vi "LIDAR Debug Platform.vi"() -> ()   [LabVIEW 2009]
uses:
  <vilib>/rvi/interface/nirviOpenFPGA/nirviOpenFPGA.xnode
  FPGA Bitfiles/Athena Brain.lvproj_FPGA Target 2_serial FPGA Main.vi.lvbitx
  serial FPGA Main.vi
  <vilib>/FPGAPlugInAG/sbRIO-9642/nirviIntfOpen_sbRIO-9642.vi
  <vilib>/rvi/interface/nirviMethod/nirviMethod.xnode
  <vilib>/rvi/interface/common/niFpgaNodeNameForErrorReporting.ctl
  <vilib>/rvi/errors/niLvFpgaWhatHappensToTopLevelVI.ctl
  <vilib>/Utility/error.llb/Error Cluster From Error Code.vi
  <vilib>/RVI Host/nirviSupport.llb/nirviErrorClusterFromErrorCode.vi
  <vilib>/LabVIEW Targets/FPGA/RIO/nirio_HostInterface/nirio_EnableInterrupts.vi
  <vilib>/rvi/errors/niLvFpgaReportInternalErrorWithAdditionalInfo.vi
  <vilib>/rvi/errors/niLvFpgaAdjustHostInterfaceError.vi
  FPGA/behaviors/driveable path/drivable paths global.vi
  <vilib>/userDefined/High Color/nirio_resource_hc.ctl
  NiRioSrv.dll
  <vilib>/rvi/FIFO/Fifo_Resource/nirvififoUniquifyingName.vi
  <vilib>/rvi/DataTransferAndStorage/Container/XNode/niFpgaContainer.xnode
panel:
  out "process time":u32
  out "transform":u32
  out "XY Graph":T1(graph)
  in  "write?":bool
  in  "Data to write":string="\u0002\u0000\u0002\u0000 $4\b"
  out "error out":errorcluster
  out "LIDAR String":string
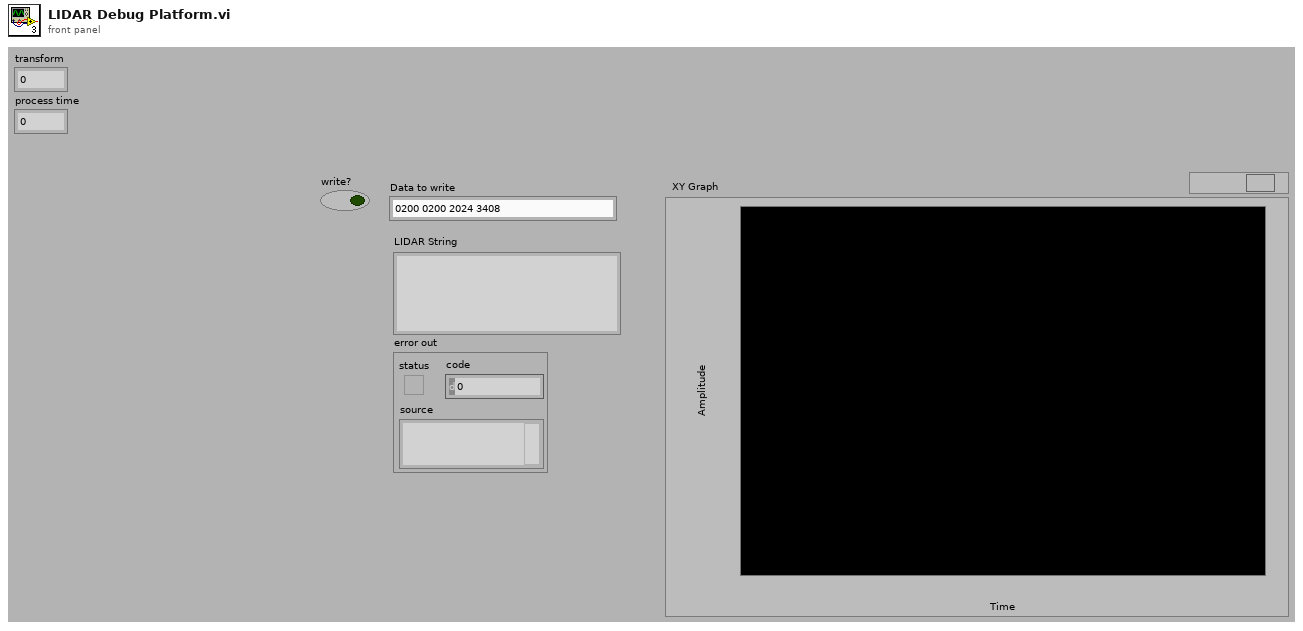
[diagram p1: front panel]
types:
  T1 = cluster{"New X Position":i16, "New Y Position":i16}[]
  T2 = typedef "serial FPGA main reference type def.ctl" = refnum<k20>
  T3 = enum16{"confirm check sum", "check status byte", "read measured values", "confirm measurement", "confirm command", "read message length", "read address", "wait for \"02\""}
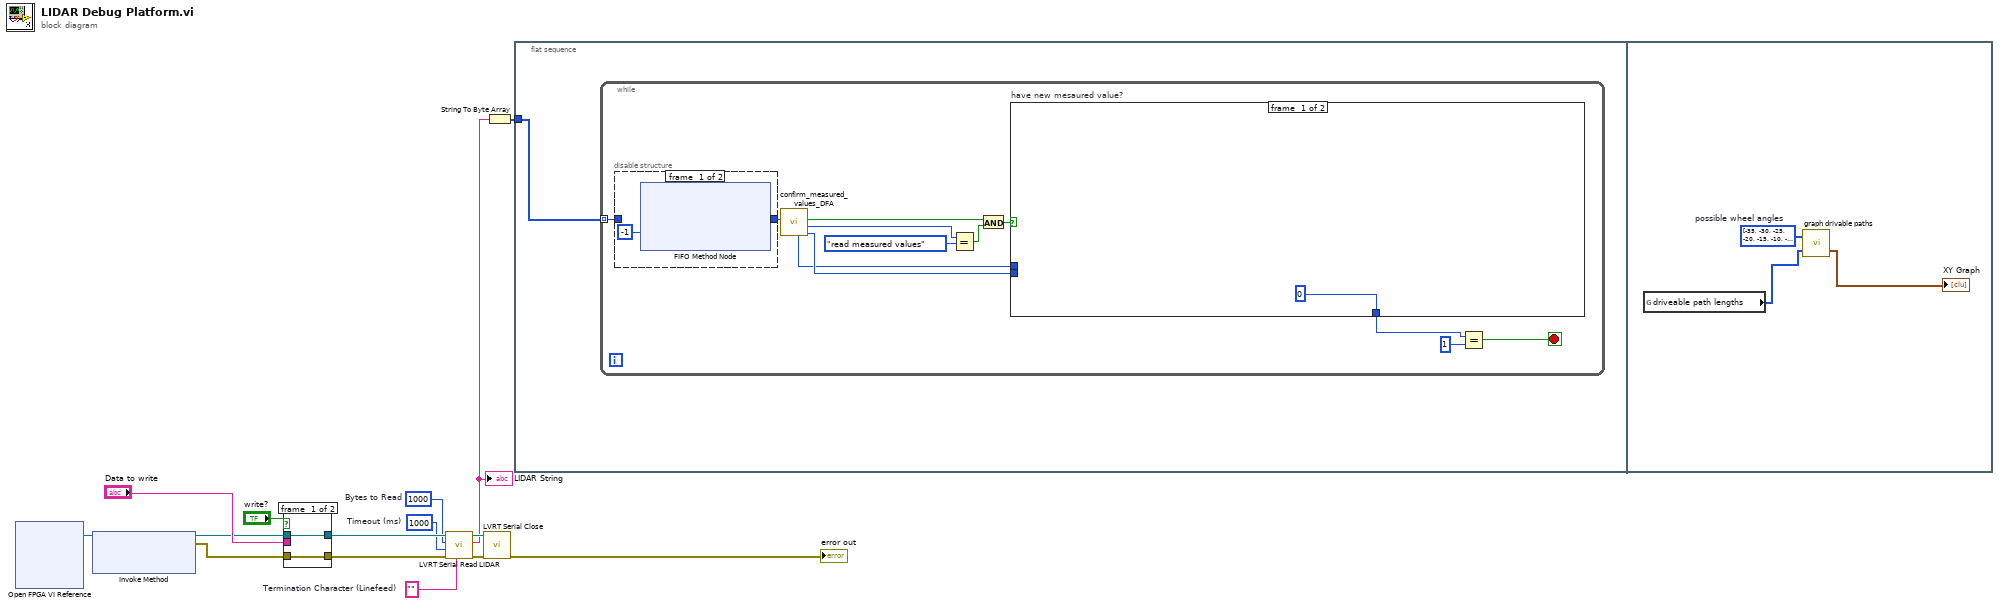
[diagram p0: block diagram]
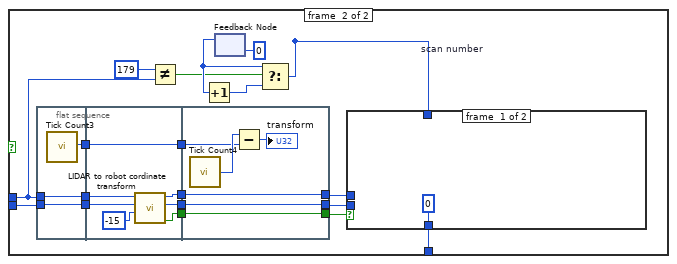
[diagram p3: hidden frame]
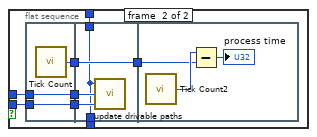
[diagram p4: hidden frame]
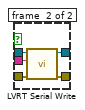
[diagram p5: hidden frame]
diagram:
  w5 = ""  # Termination Character (Linefeed)
  w10 = 1000  # Timeout (ms)
  w12 = u32 1000  # Bytes to Read
  n1 = xnode "Open FPGA VI Reference"() -> ("FPGA VI Reference Out"=w8:refnum<k20>)  [unwired: 2 in, 1 out]
  n2 = xnode "Invoke Method"("FPGA VI Reference In"=w8) -> ("FPGA VI Reference Out"=w7:refnum<k20>, "error out"=w6:errorcluster)  [unwired: 1 in, 1 out]
  n3 = case shown="False" "write?" {
    tunnel: "Data to write" -> [_ w22]
    tunnel: [w16 w21] -> w14
    tunnel: [w17 w20] -> w13
    tunnel: w7 -> [w17 w19]
    tunnel: w6 -> [w16 w18]
    frame #0 {
    }
    frame #1 {
      n4 = call "LVRT Serial Write.vi"("error in (no error)"=w18, "String"=w22, "FPGA Main Ref"=w19) -> ("error out"=w21:errorcluster, "FPGA Main Ref Out"=w20:T2)  [unwired: 7 in]
    }
  }
  n5 = call "LVRT Serial Read LIDAR.vi"("Termination Character (Linefeed)"=w5, "error in (no error)"=w14, "Timeout (ms) (-1: no timeout)"=w10, "Bytes to Read"=w12, "FPGA Main Ref"=w13) -> ("error out"=w4:errorcluster, "LIDAR"=w2:string, "FPGA Main Ref Out"=w3:T2)  [unwired: 4 in]
  "LIDAR String" <- w2
  n6 = call "LVRT Serial Close.vi"("error out"=w4, "FPGA Main Ref"=w3) -> ("error out"=→"error out":errorcluster)  [unwired: 9 out]
  n7 = String To Byte Array(string=w2) -> (unsigned byte array=w1:u8[])
  n8 = flat-sequence {
    tunnel: w1 -> [w23]
    frame #0 {
      n9 = while {
        tunnel: w23 -> [w28] mode=indexing
        stop <- w24 stop-if-true
        n10 = disable-structure shown="Enabled" {
          disable-tunnel: [w37 w86] -> w35
          disable-tunnel: w28 -> [_ w86]
          frame #0 {
            n11 = xnode ("FIFO Method Node")("Timeout"=-1) -> ("Element"=w37:u8)  [unwired: 1 in, 2 out]
          }
          frame #1 {
          }
        }
        n12 = call "confirm_measured_values_DFA.vi"("LIDAR raw data"=w35) -> ("last measured value"=w34:u16, "parser state"=w33:T3, "new value?"=w32:bool, "angle"=w26:u8)  [unwired: 7 in]
        n13 = Equal?(x=w33, y=T3."read measured values" ("parser state")) -> (x = y?=w29:bool)
        n14 = And(x=w32, y=w29) -> (x .and. y?=w31:bool)
        n15 = case "have new mesaured value?" shown="True" w31 {
          tunnel: w34 -> [_ w106]
          tunnel: w26 -> [_ w92]
          tunnel: [u8 0 ("y") w88] -> w25
          frame #0 {
          }
          frame #1 {
            n16 = flat-sequence {
              tunnel: w92 -> [w127]
              tunnel: w106 -> [w128]
              tunnel: [w128] -> w102
              tunnel: [w127] -> w101
              tunnel: [w126] -> w97
              tunnel: w102 -> [w135]
              tunnel: w101 -> [w131]
              tunnel: [w133] -> w100
              tunnel: [w132] -> w99
              tunnel: [w130] -> w98
              tunnel: w97 -> [w129]
              tunnel: [w129] -> w96
              tunnel: [w139] -> w103
              tunnel: [w140] -> w104
              tunnel: [w141] -> w105
              tunnel: w100 -> [w141]
              tunnel: w99 -> [w140]
              tunnel: w98 -> [w139]
              tunnel: w96 -> [w137]
              frame #0 {
                n17 = call "Tick Count3"() -> ("Tick Count(Ticks)"=w126:u32)
              }
              frame #1 {
                n18 = call "LIDAR to robot cordinate transform.vi"("Lidar Vertical Position"=i8 -15, "Lidar Distance"=w135, "Lidar Scan Angle"=w131) -> ("Is object?"=w130:bool, "Robot Y"=w132:i16, "Lidar X = Robot X"=w133:i16)  [unwired: 3 in, 3 out]
              }
              frame #2 {
                n19 = call "Tick Count4"() -> ("Tick Count(Ticks)"=w138:u32)
                n20 = Subtract(x=w138, y=w137) -> (x-y=→"transform":u32)
              }
            }
            n21 = Not Equal?(x=u8 179, y=w92) -> (x != y?=w93:bool)
            n22 = feedback #1 "scan number"(u8 0 ("y")) -> (w95:u8)
            n23 = Increment(x=w95) -> (x+1=w94:u8)
            n24 = Select(t=w95, s=w93, f=w94) -> (s? t:f=w90:u8)
            n25 = case shown="True" w103 {
              tunnel: w105 -> [_ w115]
              tunnel: w104 -> [_ w114]
              tunnel: w90 -> [_ w109]
              tunnel: [u8 0 ("y") w108] -> w88
              frame #0 {
              }
              frame #1 {
                n26 = flat-sequence {
                  tunnel: w114 -> [w117]
                  tunnel: w115 -> [w118]
                  tunnel: [w118] -> w113
                  tunnel: [w117] -> w112
                  tunnel: [w116] -> w111
                  tunnel: w113 -> [w122]
                  tunnel: w112 -> [w121]
                  tunnel: w111 -> [w120]
                  tunnel: [w120] -> w110
                  tunnel: w109 -> [w119]
                  tunnel: [w119] -> w108
                  tunnel: w110 -> [w124]
                  frame #0 {
                    n27 = call "Tick Count"() -> ("Tick Count(Ticks)"=w116:u32)
                  }
                  frame #1 {
                    n28 = call "update drivable paths.vi"("Robot Y"=w121, "Robot X"=w122, "Scan Number"=w119) -> ()  [unwired: 3 in]
                  }
                  frame #2 {
                    n29 = call "Tick Count2"() -> ("Tick Count(Ticks)"=w125:u32)
                    n30 = Subtract(x=w125, y=w124) -> (x-y=→"process time":u32)
                  }
                }
              }
            }
          }
        }
        n31 = Equal?(x=w25, y=u8 1) -> (x = y?=w24:bool)
      }
    }
    frame #1 {
      w144 = i8[] [-35, -30, -25, -20, -15, -10, -5, -1, 1, 5, 10, 15, 20, 25, 30, 35]  # possible wheel angles
      n32 = global read "drivable paths global.vi" "driveable path lengths"() -> (w142:u16[])
      n33 = call "graph drivable paths.vi"("updated max path lengths"=w142, "possible wheel angles"=w144) -> ("XY Graph"=→"XY Graph":T1)  [unwired: 1 in]
    }
  }
